vi "TimeTable_Panel.vi"(8 "error in (no error)":errorcluster, 11 "PanelController":refnum<class "MemberPanel.lvclass">) -> (0 "error out":errorcluster, 3 "MemberTable.lvclass":refnum<class "TimeTable.lvclass">)   [LabVIEW 2015, in "Member_Actor.lvlib"]
uses:
  Member_Actor.lvlib
  MemberTable/TimeTable.lvclass
  MemberPanel/MemberPanel.lvclass
  <vilib>/Utility/error.llb/Error Cluster From Error Code.vi
  <vilib>/ErrorRing/Error Ring.xnode
panel:
  in  "修改课程表":bool
  in  "课程表":cluster{"结束周":dbl, "起始周":dbl, "课程名称":string}[][](array[cluster])
  in  "Stop":bool
  # "—"
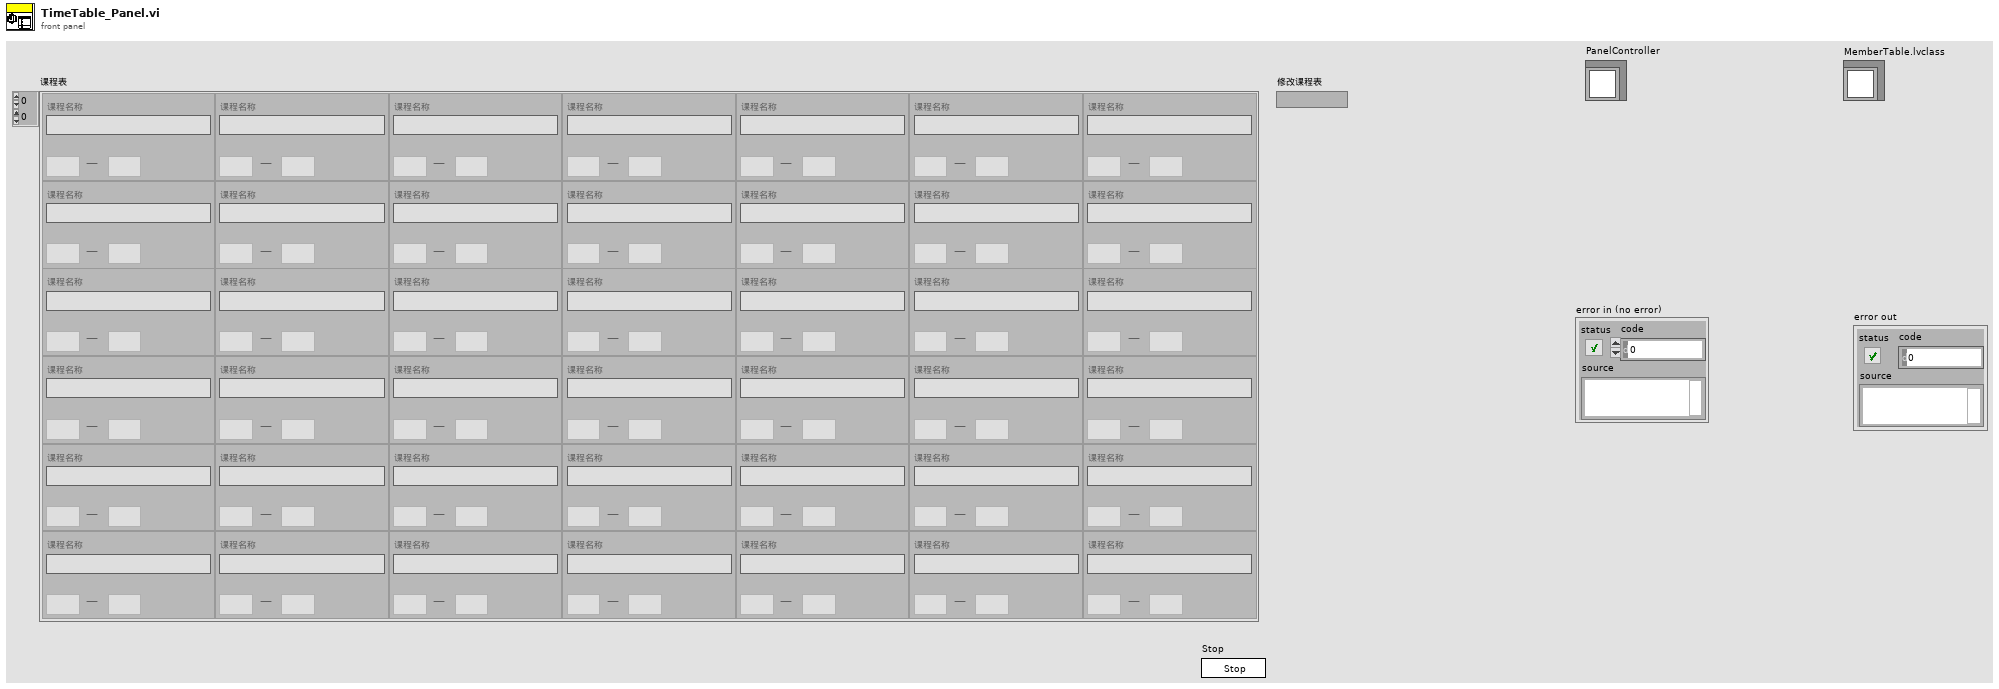
[diagram p1: front panel]
types:
  T1 = enum32{"Invalid", "Standard", "Closed", "Hidden", "Minimized", "Maximized"}
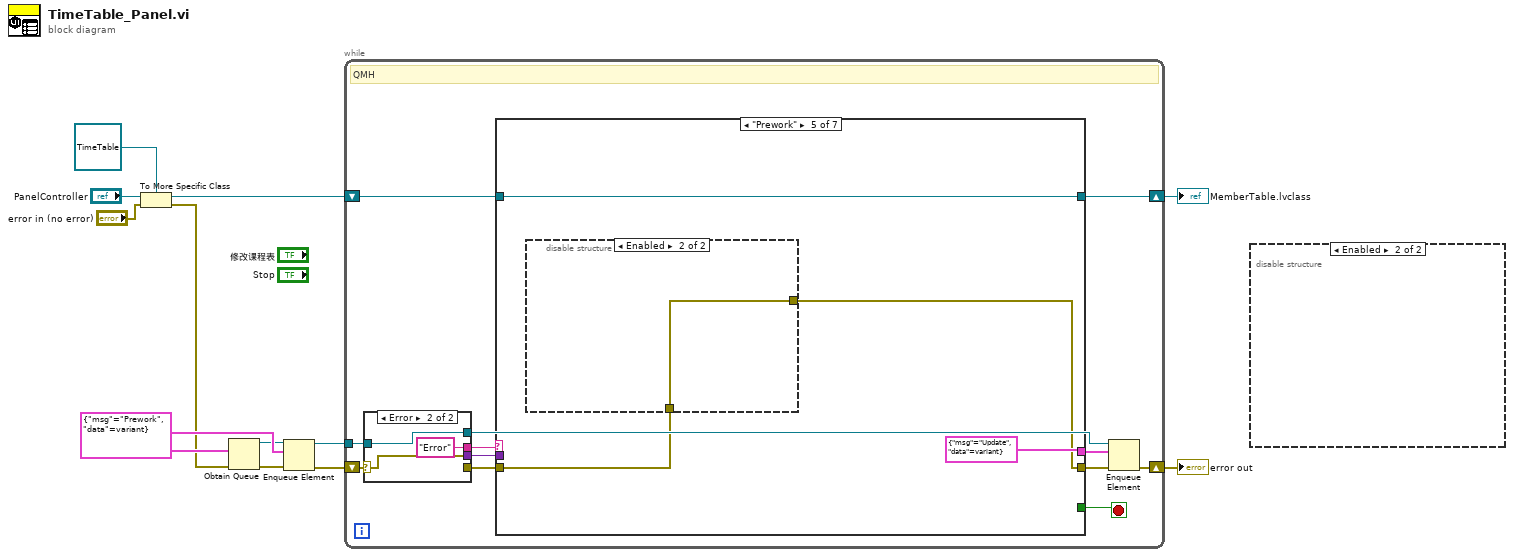
[diagram p0: block diagram]
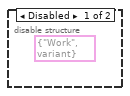
[diagram p2: hidden frame]
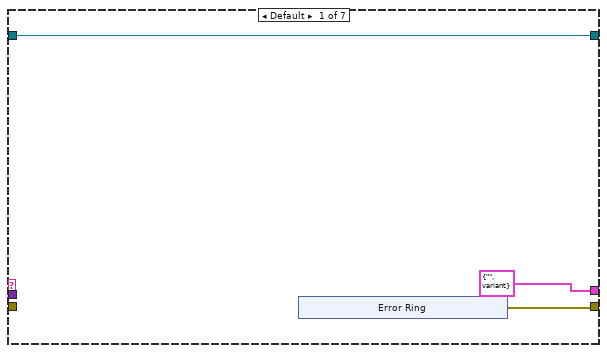
[diagram p3: hidden frame]
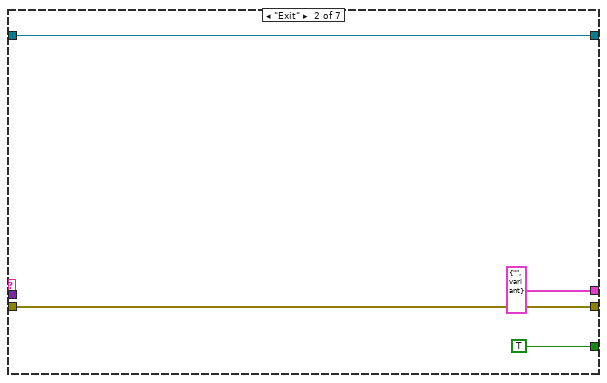
[diagram p4: hidden frame]
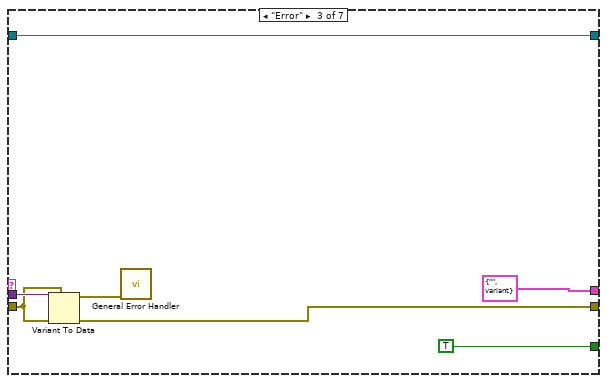
[diagram p5: hidden frame]
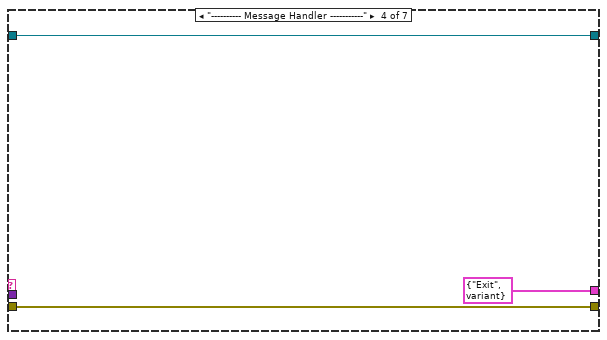
[diagram p6: hidden frame]
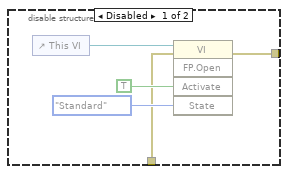
[diagram p7: hidden frame]
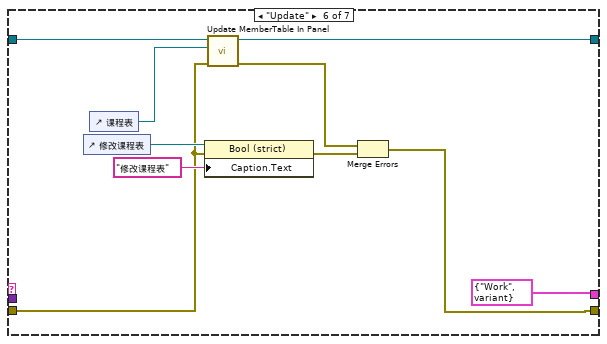
[diagram p8: hidden frame]
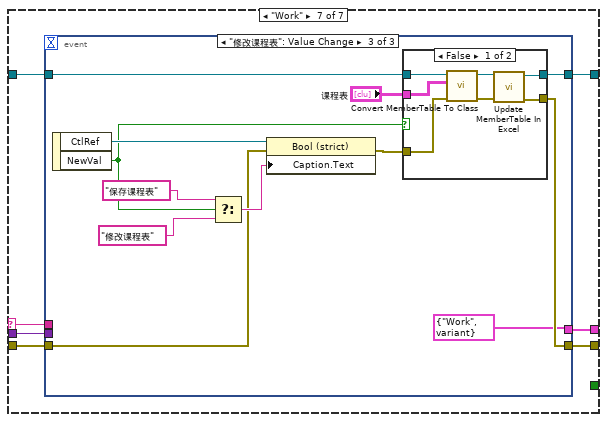
[diagram p9: hidden frame]
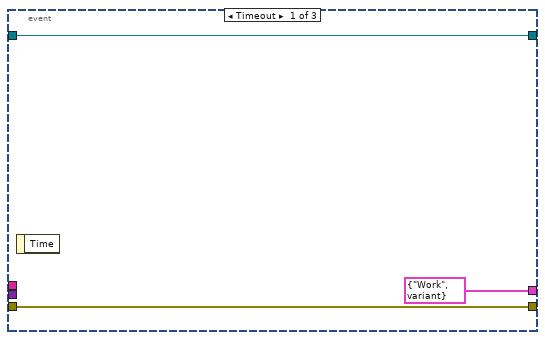
[diagram p10: hidden frame]
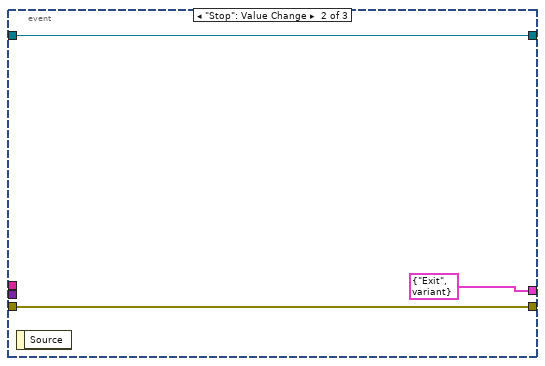
[diagram p11: hidden frame]
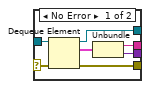
[diagram p13: hidden frame]
diagram:
  w10 = cluster{"msg":string, "data":variant} {"msg"="Prework", "data"=variant}
  n1 = To More Specific Class(target class=refnum<class "TimeTable.lvclass"> refnum ("MemberTable.lvclass"), reference="PanelController", error in="error in (no error)") -> (specific class reference=w3:refnum<class "TimeTable.lvclass">, error out=w1:errorcluster)
  n2 = Obtain Queue(element data type=w10, error in (no error)=w1) -> (queue out=w8:refnum<queue>, error out=w9:errorcluster)  [unwired: 3 in, 1 out]
  n3 = Enqueue Element(queue=w8, element=w10, error in (no error)=w9) -> (queue out=w11:refnum<queue>, error out=w12:errorcluster)  [unwired: 1 in, 1 out]
  n4 = while {
    tunnel: w11 -> [w23]
    shift-right: [w18] -> w6
    shift-left: w12 -> [w24]
    shift-right: [w13] -> w7
    shift-left: w3 -> [w14]
    stop <- w15 stop-if-true
    # "QMH"
    n5 = case shown="Error" w24 {
      selector: w24 -> [w106 w110]
      tunnel: w23 -> [w107 w108]
      tunnel: [w105 _] -> w22
      tunnel: [w103 "Error" ("msg")] -> w21
      tunnel: [w102 w110] -> w20
      tunnel: [w101 w108] -> w17
      frame No Error {
        n6 = Dequeue Element(queue=w107, error in (no error)=w106) -> (queue out=w101:refnum<queue>, element=w104:cluster{"msg":string, "data":variant}, error out=w105:errorcluster)  [unwired: 1 in, 1 out]
        n7 = Unbundle(w104) -> ("msg"=w103:string, "data"=w102:variant)
      }
      frame Error {
      }
    }
    n8 = case shown="\"Prework\"" w21 {
      selector: w21 -> [_ _ _ _ _ _ w71]
      tunnel: w22 -> [_ w36 w42 w46 w48 w61 w73]
      tunnel: w20 -> [_ _ w43 _ _ _ w72]
      tunnel: [w27 w36 w40 w46 w47 w58 w70] -> w19
      tunnel: [cluster{"msg":string, "data":variant} {"msg"="", "data"=variant} cluster{"msg":string, "data":variant} {"msg"="", "data"=variant} cluster{"msg":string, "data":variant} {"msg"="", "data"=variant} cluster{"msg":string, "data":variant} {"msg"="Exit", "data"=variant} cluster{"msg":string, "data":variant} {"msg"="Update", "data"=variant} cluster{"msg":string, "data":variant} {"msg"="Work", "data"=variant} w69] -> w16
      tunnel: [_ TRUE TRUE _ _ _ _] -> w15
      tunnel: w14 -> [w25 w33 w37 w44 w49 w65 w68]
      tunnel: [w25 w33 w37 w44 w49 w57 w67] -> w13
      frame Default {
        n9 = xnode "Error Ring"() -> ("error out"=w27:errorcluster)
      }
      frame "Exit" {
      }
      frame "Error" {
        n10 = Variant To Data(error in=w42, type=w42, Variant=w43) -> (data=w41:errorcluster, error out=w40:errorcluster)
        n11 = call <vilib>:"General Error Handler.vi"("error in (no error)"=w41) -> ()  [unwired: 10 in, 5 out]
      }
      frame "---------- Message Handler -----------" {
      }
      frame "Prework" {
        n12 = disable-structure shown="Enabled" {
          disable-tunnel: w48 -> [w52 w56]
          disable-tunnel: [w51 w56] -> w47
          frame Disabled {
            n13 = control-ref of="This VI"() -> (w55:refnum<vi>)
            n14 = invoke class="VI" method="FP.Open"(reference=w55, error in=w52, "Activate"=TRUE ("Activate?"), "State"=T1."Standard") -> (error out=w51:errorcluster)  [unwired: 1 in, 4 out]
          }
          frame Enabled {
          }
        }
      }
      frame "Update" {
        n15 = control-ref of="修改课程表"() -> (w63:refnum<vi>)
        n16 = control-ref of="课程表"() -> (w64:refnum<vi>)
        n17 = property class="Bool (strict)"(reference=w63, error in=w61, "Caption.Text"="修改课程表") -> (error out=w60:errorcluster)  [unwired: 1 out]
        n18 = call "Update MemberTable In Panel.vi"("error in (no error)"=w61, "课程表"=w64, "MemberTable in"=w65) -> ("error out"=w59:errorcluster, "MemberTable out"=w57:refnum<class "TimeTable.lvclass">)  [unwired: 7 in]
        n19 = Merge Errors(w59, w60) -> (w58:errorcluster)
      }
      frame "Work" {
        n20 = event shown="[2] \"修改课程表\": Value Change" {
          selector: _ -> [_ _ _]
          dyn-events: _ -> [_ _ _]
          timeout: _ -> [_ _ _]
          tunnel: w73 -> [w76 w79 w87]
          tunnel: w72 -> [_ _ _]
          tunnel: w71 -> [_ _ _]
          tunnel: [w76 w79 w81] -> w70
          tunnel: [cluster{"msg":string, "data":variant} {"msg"="Work", "data"=variant} cluster{"msg":string, "data":variant} {"msg"="Exit", "data"=variant} cluster{"msg":string, "data":variant} {"msg"="Work", "data"=variant}] -> w69
          tunnel: w68 -> [w74 w77 w85]
          tunnel: [w74 w77 w82] -> w67
          event Timeout {
            n21 = event-data() -> ()  [unwired: 1 in, 1 out]
          }
          event "Stop": Value Change {
            n22 = event-data() -> ()  [unwired: 1 in, 1 out]
          }
          event "修改课程表": Value Change {
            n23 = event-data() -> ("CtlRef"=w89:refnum<vi>, "NewVal"=w86:bool)  [unwired: 1 in]
            n24 = Select(t="保存课程表", s=w86, f="修改课程表") -> (s? t:f=w88:string)
            n25 = property class="Bool (strict)"(reference=w89, error in=w87, "Caption.Text"=w88) -> (error out=w83:errorcluster)  [unwired: 1 out]
            n26 = case shown="False" w86 {
              tunnel: w85 -> [w98 w100]
              tunnel: "课程表" -> [w97 _]
              tunnel: w83 -> [w96 w99]
              tunnel: [w93 w100] -> w82
              tunnel: [w92 w99] -> w81
              frame False {
                n27 = call "Convert MemberTable To Class.vi"("error in (no error)"=w96, "课程表"=w97, "MemberTable in"=w98) -> ("error out"=w94:errorcluster, "MemberTable out"=w95:refnum<class "TimeTable.lvclass">)  [unwired: 7 in]
                n28 = call "Update MemberTable In Excel.vi"("error in (no error)"=w94, "MemberTable in"=w95) -> ("error out"=w92:errorcluster, "MemberTable out"=w93:refnum<class "TimeTable.lvclass">)  [unwired: 8 in]
              }
              frame True {
              }
            }
          }
        }
      }
    }
    n29 = Enqueue Element(queue=w17, element=w16, error in (no error)=w19) -> (error out=w18:errorcluster)  [unwired: 1 in, 2 out]
  }
  "MemberTable.lvclass" <- w7
  "error out" <- w6
  n30 = disable-structure shown="Enabled" {
    frame Disabled {
      (unwired) cluster{"msg":string, "data":variant} {"msg"="Work", "data"=variant}
    }
    frame Enabled {
    }
  }
